vi "Simple_Test.vi"(8 "error in":errorcluster, 11 "Powermeter_COMPort":refnum<visa-resource-name>="USB0::0x1313::0x8078::PM001523::INSTR" caption="instrument handle") -> (0 "error out":errorcluster, 3 "Power":dbl)   [LabVIEW 2024]
panel:
  in  "STOP":bool
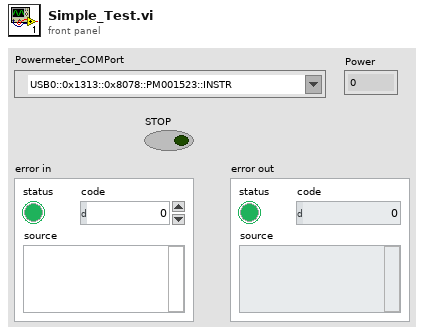
[diagram p1: front panel]
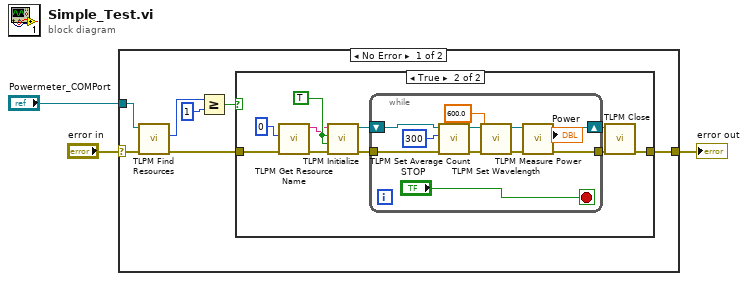
[diagram p0: block diagram]
diagram:
  n1 = case shown="No Error" "error in" {
    selector: "error in" -> [w10 w34]
    tunnel: [w4 w34] -> w2
    tunnel: "Powermeter_COMPort" -> [w9 _]
    frame No Error {
      n2 = call <instrlib>:"TLPM Find Resources.vi"("error in (no error)"=w10, "instrument handle"=w9) -> ("error out"=w6:errorcluster, "Resource Count"=w7:u32)  [unwired: 7 in, 1 out]
      n3 = Greater Or Equal?(x=w7, y=u32 1) -> (x >= y?=w5:bool)
      n4 = case shown="True" w5 {
        tunnel: w6 -> [w11 w19]
        tunnel: [w11 w13] -> w4
        frame False {
        }
        frame True {
          w18 = TRUE ("ID Query (Do Query)")
          n5 = call <instrlib>:"TLPM Get Resource Name.vi"("error in (no error)"=w19, "Index (0)"=u32 0 ("Device Index")) -> ("error out"=w21:errorcluster, "Resource Name"=w12:string)  [unwired: 7 in, 1 out]
          n6 = call <instrlib>:"TLPM Initialize.vi"("error in (no error)"=w21, "Reset Device (Reset Device)"=w18, "ID Query (Do Query)"=w18, "resource name"=w12) -> ("error out"=w16:errorcluster, "instrument handle out"=w17:refnum<visa-resource-name>)  [unwired: 6 in]
          n7 = while {
            shift-right: [w27] -> w14
            shift-left: w17 -> [w32]
            tunnel: [w26] -> w15
            tunnel: w16 -> [w25]
            stop <- "STOP" stop-if-true
            n8 = call <instrlib>:"TLPM Set Average Count.vi"("error in (no error)"=w25, "Average Count (1)"=i16 300, "instrument handle"=w32) -> ("error out"=w30:errorcluster, "instrument handle out"=w31:refnum<visa-resource-name>)  [unwired: 7 in]
            n9 = call <instrlib>:"TLPM Set Wavelength.vi"("error in (no error)"=w30, "Wavelength (0.0)"=600.0, "instrument handle"=w31) -> ("error out"=w29:errorcluster, "instrument handle out"=w28:refnum<visa-resource-name>)  [unwired: 7 in]
            n10 = call <instrlib>:"TLPM Measure Power.vi"("error in (no error)"=w29, "instrument handle"=w28) -> ("error out"=w26:errorcluster, "Power"=→"Power":dbl, "instrument handle out"=w27:refnum<visa-resource-name>)  [unwired: 7 in]
          }
          n11 = call <instrlib>:"TLPM Close.vi"("error in (no error)"=w15, "instrument handle"=w14) -> ("error out"=w13:errorcluster)  [unwired: 9 in]
        }
      }
    }
    frame Error {
    }
  }
  "error out" <- w2
